vi "SetOutput.vi"(8 "error in (no error)":errorcluster, 9 "Boolean":bool=TRUE, 10 "Index":i32, 11 "ZanCard in":refnum<class "ZanCard.lvclass">) -> (0 "error out":errorcluster, 1 "life+1":bool, 3 "ZanCard out":refnum<class "ZanCard.lvclass">)   [LabVIEW 2019, in "ZanCard.lvclass"]
uses:
  ZanCard.lvclass
  ZanCard.lvclass/ZanCard.ctl
  LLB/zmotion/zaux/zauxdll.lvlib
panel:
  out "Index":i32
  out "OutData":bool[](array[boolean])
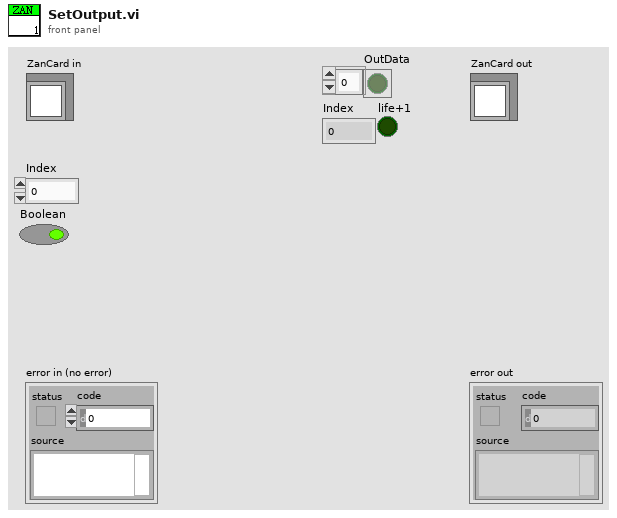
[diagram p1: front panel]
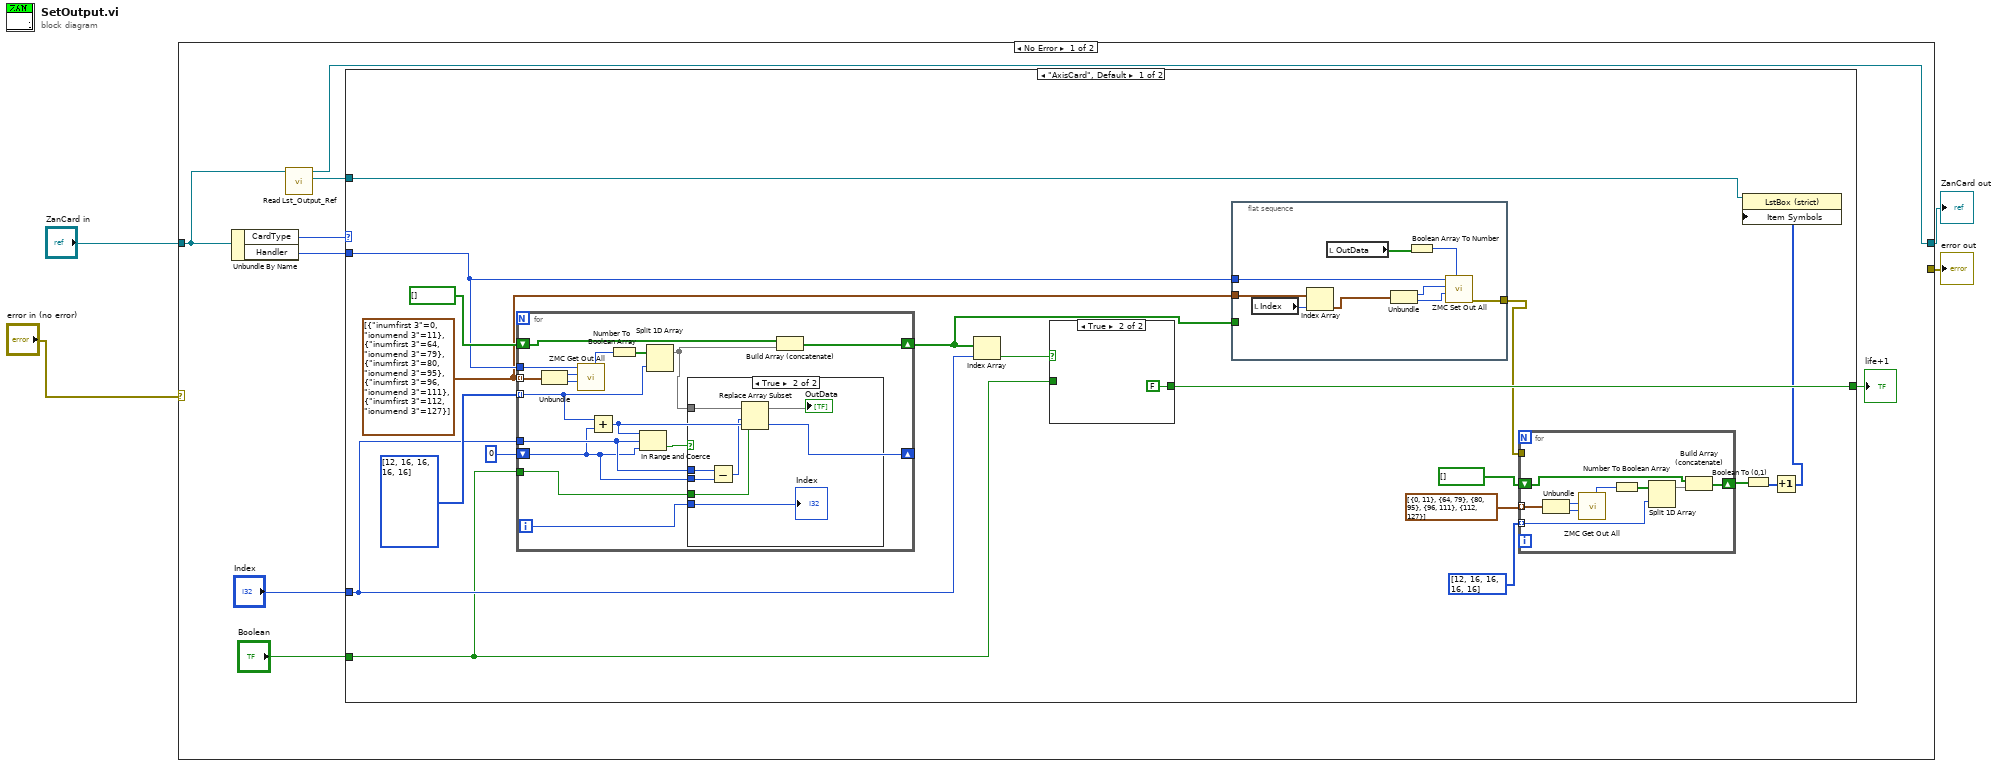
[diagram p0: block diagram]
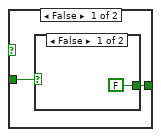
[diagram p2: hidden frame]
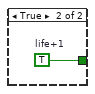
[diagram p3: hidden frame]
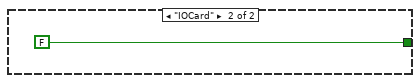
[diagram p5: hidden frame]
diagram:
  n1 = case shown="No Error" "error in (no error)" {
    selector: "error in (no error)" -> [_ w79]
    tunnel: "ZanCard in" -> [w7 w78]
    tunnel: [_ w79] -> w2
    tunnel: [w5 w78] -> w1
    frame No Error {
      n2 = Unbundle By Name(w7) -> ("CardType"=w11:enum16{"AxisCard", "IOCard"}, "Handler"=w12:i32)
      n3 = call-dynamic "Read Lst_Output_Ref.vi"("IOCard in"=w7) -> ("Lst_Output_Ref"=w6:refnum<vi>, "IOCard out"=w5:refnum<class "ZanCard.lvclass">)  [unwired: 8 in, 1 out]
      n4 = case shown="\"AxisCard\", Default" w11 {
        tunnel: w12 -> [w26 _]
        tunnel: "Index" -> [w24 _]
        tunnel: "Boolean" -> [w23 _]
        tunnel: [w27 FALSE ("life+1")] -> w8
        tunnel: w6 -> [w16 _]
        frame "AxisCard", Default {
          w22 = cluster{"inumfirst 3":u16, "ionumend 3":i32}[] [{"inumfirst 3"=0, "ionumend 3"=11}, {"inumfirst 3"=64, "ionumend 3"=79}, {"inumfirst 3"=80, "ionumend 3"=95}, {"inumfirst 3"=96, "ionumend 3"=111}, {"inumfirst 3"=112, "ionumend 3"=127}]
          n5 = for {
            tunnel: w26 -> [w69]
            tunnel: w22 -> [w68] mode=indexing
            shift-right: [w65] -> w21
            shift-left: bool[] [] -> [w63]
            tunnel: u16[] [12, 16, 16, 16, 16] -> [w61] mode=indexing
            tunnel: w24 -> [w57]
            shift-right: [w60] -> _
            shift-left: 0 -> [w56]
            tunnel: w23 -> [w55]
            i -> [w54]
            n6 = Unbundle(w68) -> ("inumfirst 3"=w67:u16, "ionumend 3"=w66:i32)
            n7 = call "ZMC Get Out All.vi"("inumend"=w66, "inumfirst"=w67, "handle"=w69) -> ("pistate out"=w64:u32)  [unwired: 5 in, 3 out]
            n8 = Add(x=w61, y=w56) -> (x+y=w60:i32)
            n9 = Number To Boolean Array(number=w64) -> (Boolean array=w62:bool[])
            n10 = In Range and Coerce(upper limit=w60, x=w57, lower limit=w56) -> (In Range?=w59:bool)  [unwired: 1 out]
            n11 = Split 1D Array(array=w62, index=w61) -> (first subarray=w58:bool[])  [unwired: 1 out]
            n12 = case shown="True" w59 {
              tunnel: w58 -> [_ w76]
              tunnel: w57 -> [_ w75]
              tunnel: w56 -> [_ w74]
              tunnel: w55 -> [_ w72]
              tunnel: w54 -> [_ w70]
              frame False {
              }
              frame True {
                n13 = Subtract(x=w75, y=w74) -> (x-y=w73:i32)
                n14 = Replace Array Subset(array=w76, new element=w72, index=w73) -> (→"OutData":bool[])
                "Index" <- w70
              }
            }
            n15 = Build Array (concatenate)(w63, w58) -> (w65:bool[])
          }
          n16 = Index Array(array=w21, index=w24) -> (element=w28:bool)
          n17 = case shown="True" w28 {
            tunnel: w23 -> [w50 _]
            tunnel: [w49 FALSE ("life+1")] -> w27
            frame False {
              n18 = case shown="False" w50 {
                tunnel: [FALSE ("life+1") w52] -> w49
                frame False {
                }
                frame True {
                  w52 = TRUE  # life+1
                }
              }
            }
            frame True {
            }
          }
          n19 = flat-sequence {
            tunnel: w26 -> [w48]
            tunnel: w22 -> [w46]
            tunnel: w21 -> [_]
            tunnel: [w40] -> w17
            frame #0 {
              n20 = local read "Index"() -> (w44:i32)
              n21 = Index Array(array=w46, index=w44) -> (element=w43:cluster{"inumfirst 3":u16, "ionumend 3":i32})
              n22 = local read "OutData"() -> (w45:bool[])
              n23 = Unbundle(w43) -> ("inumfirst 3"=w42:u16, "ionumend 3"=w41:i32)
              n24 = Boolean Array To Number(Boolean array=w45) -> (number=w47:u32)
              n25 = call "ZMC Set Out All.vi"("istate"=w47, "inumend"=w41, "inumfirst"=w42, "handle"=w48) -> ("error out"=w40:errorcluster)  [unwired: 5 in, 2 out]
            }
          }
          n26 = for {
            tunnel: cluster{"inumfirst 3":u16, "ionumend 3":i32}[] [{"inumfirst 3"=0, "ionumend 3"=11}, {"inumfirst 3"=64, "ionumend 3"=79}, {"inumfirst 3"=80, "ionumend 3"=95}, {"inumfirst 3"=96, "ionumend 3"=111}, {"inumfirst 3"=112, "ionumend 3"=127}] -> [w39] mode=indexing
            shift-right: [w36] -> w15
            shift-left: bool[] [] -> [w34]
            tunnel: u16[] [12, 16, 16, 16, 16] -> [w32] mode=indexing
            tunnel: w17 -> [_]
            n27 = Unbundle(w39) -> ("inumfirst 3"=w38:u16, "ionumend 3"=w37:i32)
            n28 = call "ZMC Get Out All.vi"("inumend"=w37, "inumfirst"=w38) -> ("pistate out"=w35:u32)  [unwired: 6 in, 3 out]
            n29 = Number To Boolean Array(number=w35) -> (Boolean array=w33:bool[])
            n30 = Split 1D Array(array=w33, index=w32) -> (first subarray=w31:bool[])  [unwired: 1 out]
            n31 = Build Array (concatenate)(w34, w31) -> (w36:bool[])
          }
          n32 = Boolean To (0,1)(Boolean=w15) -> (0, 1=w14:i16[])
          n33 = Increment(x=w14) -> (x+1=w13:i16[])
          n34 = property class="LstBox (strict)"(reference=w16, "Item Symbols"=w13) -> ()  [unwired: 1 in, 2 out]
        }
        frame "IOCard" {
        }
      }
      "life+1" <- w8
    }
    frame Error {
    }
  }
  "error out" <- w2
  "ZanCard out" <- w1
